vi "Open UDP connection.vi"() -> ()   [LabVIEW 2017]
panel:
  out "error out":errorcluster
  out "connection ID":refnum<k16>
  in  "error in (no error)":errorcluster
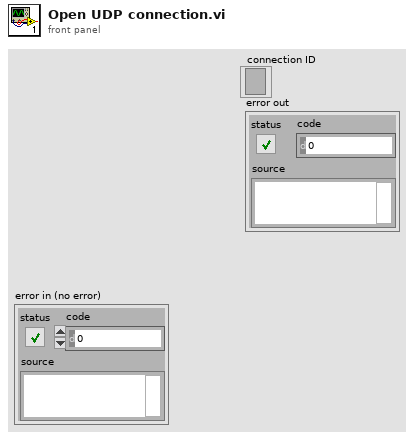
[diagram p1: front panel]
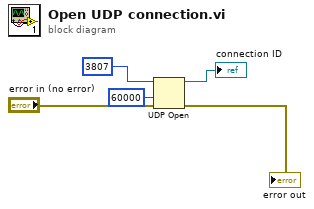
[diagram p0: block diagram]
diagram:
  n1 = UDP Open(8:"error in (no error)", 9:60000 ("timeout ms (25000)"), 11:u16 3807 ("port")) -> (port=→"connection ID":refnum<k16>, 0:→"error out":errorcluster)  [unwired: 2 in, 1 out]
